vi "update GUI nonlinPID tuning.vi"(10 "Supervisor in":refnum<class "Supervisor.lvclass">, 11 "Vessel in":refnum<class "Vessel.lvclass">) -> (2 "Supervisor":refnum<class "Supervisor.lvclass">)   [LabVIEW 2014]
uses:
  ROV/Vessel.lvclass
  Supervisor/Supervisor.lvclass
  <vilib>/Analysis/Matrix/Datatypes/RealMatrix.ctl
  Controller/PID Controller/Non Linear PID Controller/Non Linear PID Controller.lvclass
  Controller/PID Controller/PID Controller.lvclass
  <vilib>/Analysis/Matrix/NI_Matrix.lvlib
panel:
  out "K_P":T1
  in  "Name":string
  in  "Update KA":bool
  in  "Update KI":bool
  in  "Update KD":bool
  in  "Update KP":bool
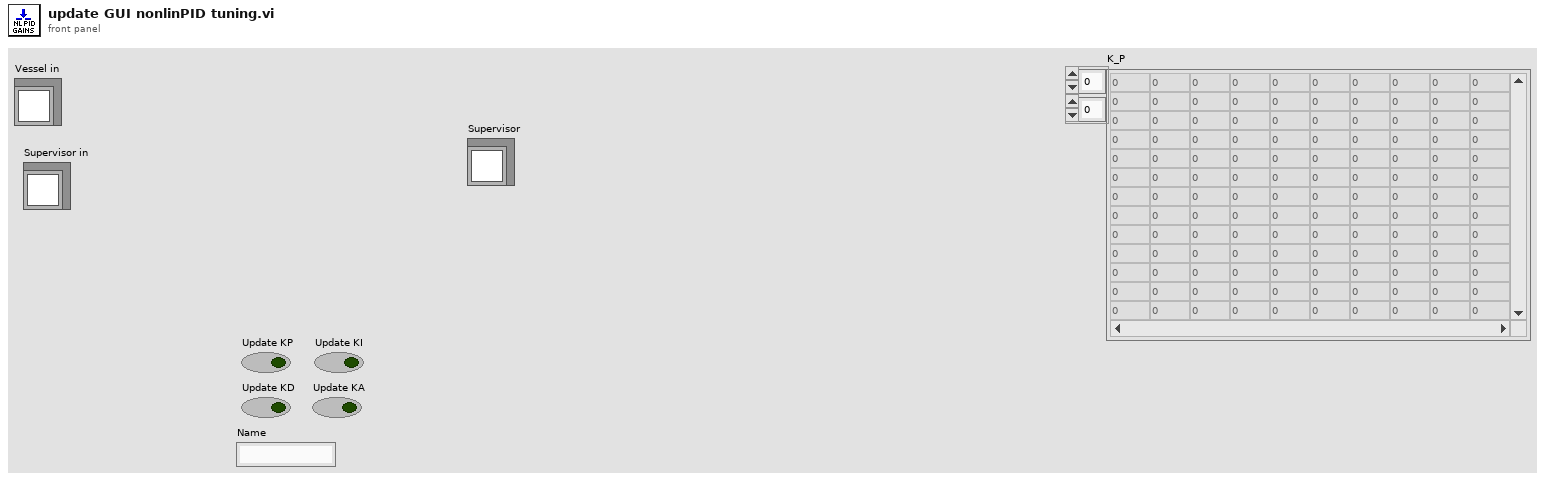
[diagram p1: front panel]
types:
  T1 = typedef "NI_Matrix.lvlib/RealMatrix.ctl" = dbl[][]
  T2 = cluster{"K_P":T1, "K_D":T1, "K_I":T1, "K_A":T1, "Update KP":bool, "Update KD":bool, "Update KI":bool, "Update KA":bool, "Name":string}
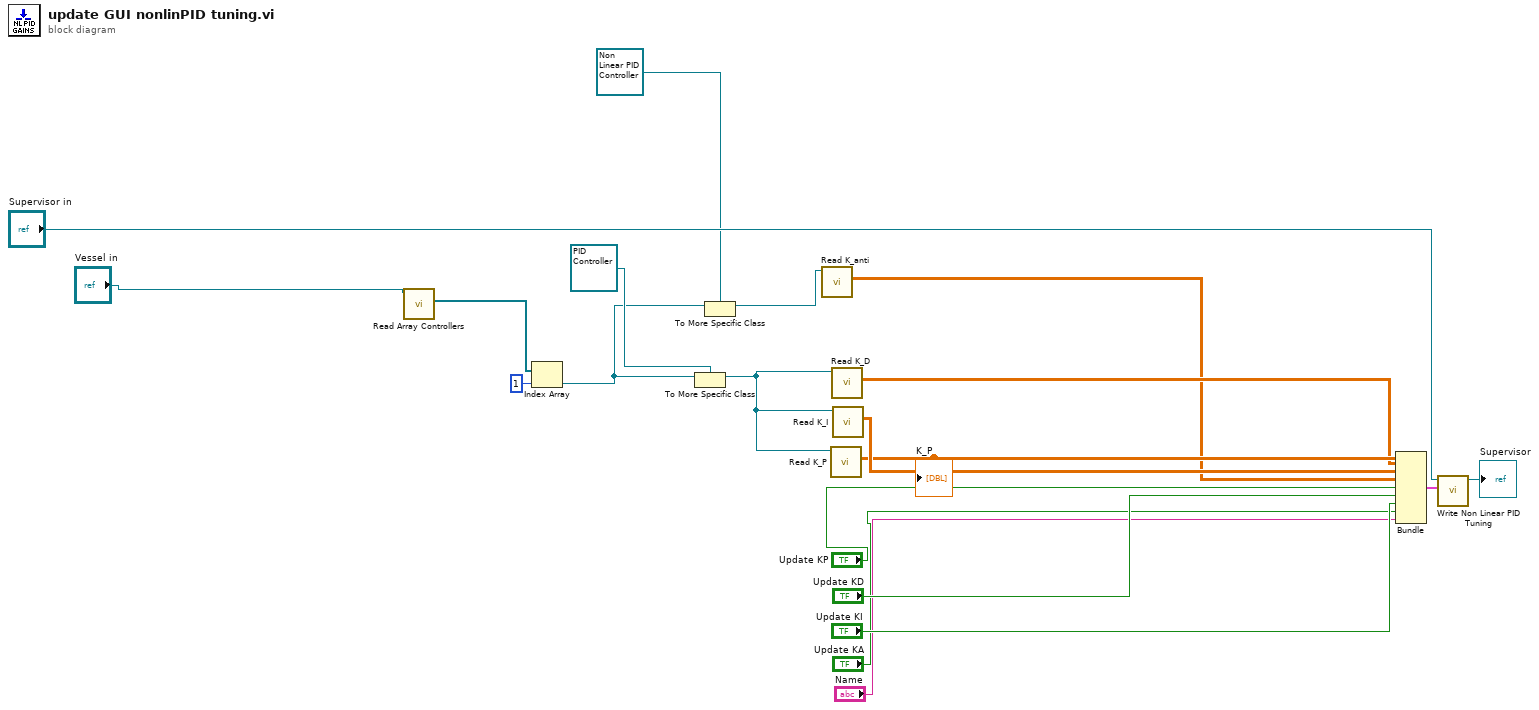
[diagram p0: block diagram]
diagram:
  n1 = call "Read Array Controllers.vi"("Vessel in"="Vessel in") -> ("Array Controllers"=w10:refnum<class "Controller.lvclass">[])  [unwired: 8 in, 2 out]
  n2 = Index Array(array=w10, index=1) -> (element=w5:refnum<class "Controller.lvclass">)
  n3 = To More Specific Class(target class=refnum<class "PID Controller.lvclass"> refnum ("Controller Library:PID Controller.lvclass"), reference=w5) -> (specific class reference=w7:refnum<class "PID Controller.lvclass">)  [unwired: 1 in, 1 out]
  n4 = To More Specific Class(target class=refnum<class "Non Linear PID Controller.lvclass"> refnum ("Controller Library:Non Linear PID Controller.lvclass"), reference=w5) -> (specific class reference=w9:refnum<class "Non Linear PID Controller.lvclass">)  [unwired: 1 in, 1 out]
  n5 = call-dynamic "Read K_anti.vi"("Non Linear PID Controller in"=w9) -> ("K_A"=w1:T1)  [unwired: 8 in, 2 out]
  n6 = call-dynamic "Read K_P.vi"("PID Controller in"=w7) -> ("K_P"=w3:T1)  [unwired: 8 in, 2 out]
  "K_P" <- w3
  n7 = call-dynamic "Read K_D.vi"("PID Controller in"=w7) -> ("K_D"=w2:T1)  [unwired: 8 in, 2 out]
  n8 = call-dynamic "Read K_I.vi"("PID Controller in"=w7) -> ("K_I"=w4:T1)  [unwired: 8 in, 2 out]
  n9 = Bundle("K_P"=w3, "K_D"=w2, "K_I"=w4, "K_A"=w1, "Update KP"="Update KP", "Update KD"="Update KD", "Update KI"="Update KI", "Update KA"="Update KA", "Name"="Name") -> (w16:T2)  [unwired: 1 in]
  n10 = call-dynamic "Write Non Linear PID Tuning.vi"("Non Linear PID Tuning"=w16, "Supervisor in"="Supervisor in") -> ("Supervisor out"=→"Supervisor":refnum<class "Supervisor.lvclass">)  [unwired: 8 in, 1 out]
